vi "RFmx_Meas_Settings_SeqMode.vi"(7 "RFmx_Setting":T1={"Center Frequency (Hz)"=0.0, "Reference Level (dBm)"=0.0, "External Attenuation (dB)"=0.0, "ACP:Offset Frequency (Hz)"=[], "ACP:Integration Bandwidth (Hz)"=[], "CCDF:Threshold Level (dB or dBm)"=0.0, "CHP:Integration Bandwidth (Hz)"=0.0, "Fcnt:Threshold Level (dB or dBm)"=0.0, "OBW:Bandwidth Percentage (%)"=0.0, "Spectrum:Span (Hz)"=20000000.0, "TXP:Measurement Interval (s)"=0.0, "IQ:Bandwidth (Hz)"=1000000.0} {"IQ:Bandwidth (Hz)" format="%#_13p"; "TXP:Measurement Interval (s)" format="%#_6p"; "Spectrum:Span (Hz)" format="%#_13p"; "OBW:Bandwidth Percentage (%)" format="%#_6p"; "Fcnt:Threshold Level (dB or dBm)" format="%#_6p"; "CHP:Integration Bandwidth (Hz)" format="%#_6p"; "CCDF:Threshold Level (dB or dBm)" format="%#_6p"; "ACP:Integration Bandwidth (Hz)" format="%#_6p"; "ACP:Offset Frequency (Hz)" format="%#_6p"; "External Attenuation (dB)" format="%#_6p"; "Reference Level (dBm)" format="%#_6p"; "Center Frequency (Hz)" format="%#_6p"}, 8 "error in":errorcluster, 9 "Selector Strings":string[](array[string]), 10 "Measurements":T2(array[ring]), 11 "Instrument Handle in":refnum<k21>) -> (0 "error out":errorcluster, 3 "Instrument Handle out":refnum<k21>)   [LabVIEW 2014]
panel:
  # "클러스터 하나로 만들어야 함"
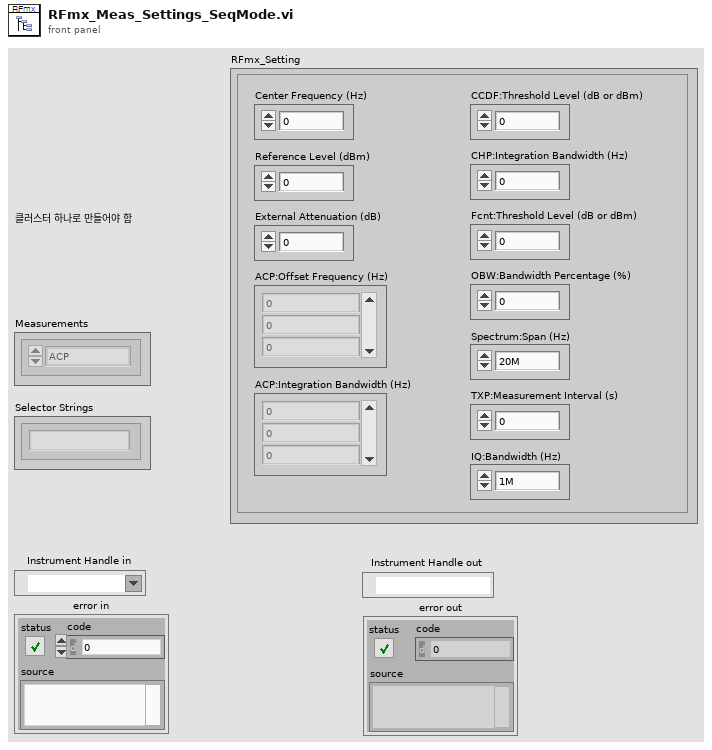
[diagram p1: front panel]
types:
  T1 = cluster{"Center Frequency (Hz)":dbl, "Reference Level (dBm)":dbl, "External Attenuation (dB)":dbl, "ACP:Offset Frequency (Hz)":dbl[], "ACP:Integration Bandwidth (Hz)":dbl[], "CCDF:Threshold Level (dB or dBm)":dbl, "CHP:Integration Bandwidth (Hz)":dbl, "Fcnt:Threshold Level (dB or dBm)":dbl, "OBW:Bandwidth Percentage (%)":dbl, "Spectrum:Span (Hz)":dbl, "TXP:Measurement Interval (s)":dbl, "IQ:Bandwidth (Hz)":dbl}
  T2 = enum16{"ACP", "CCDF", "CHP", "FCnt", "Harmonics", "OBW", "SEM", "Spectrum", "Spur", "TXP", "AMPM", "DPD", "IQ"}[]
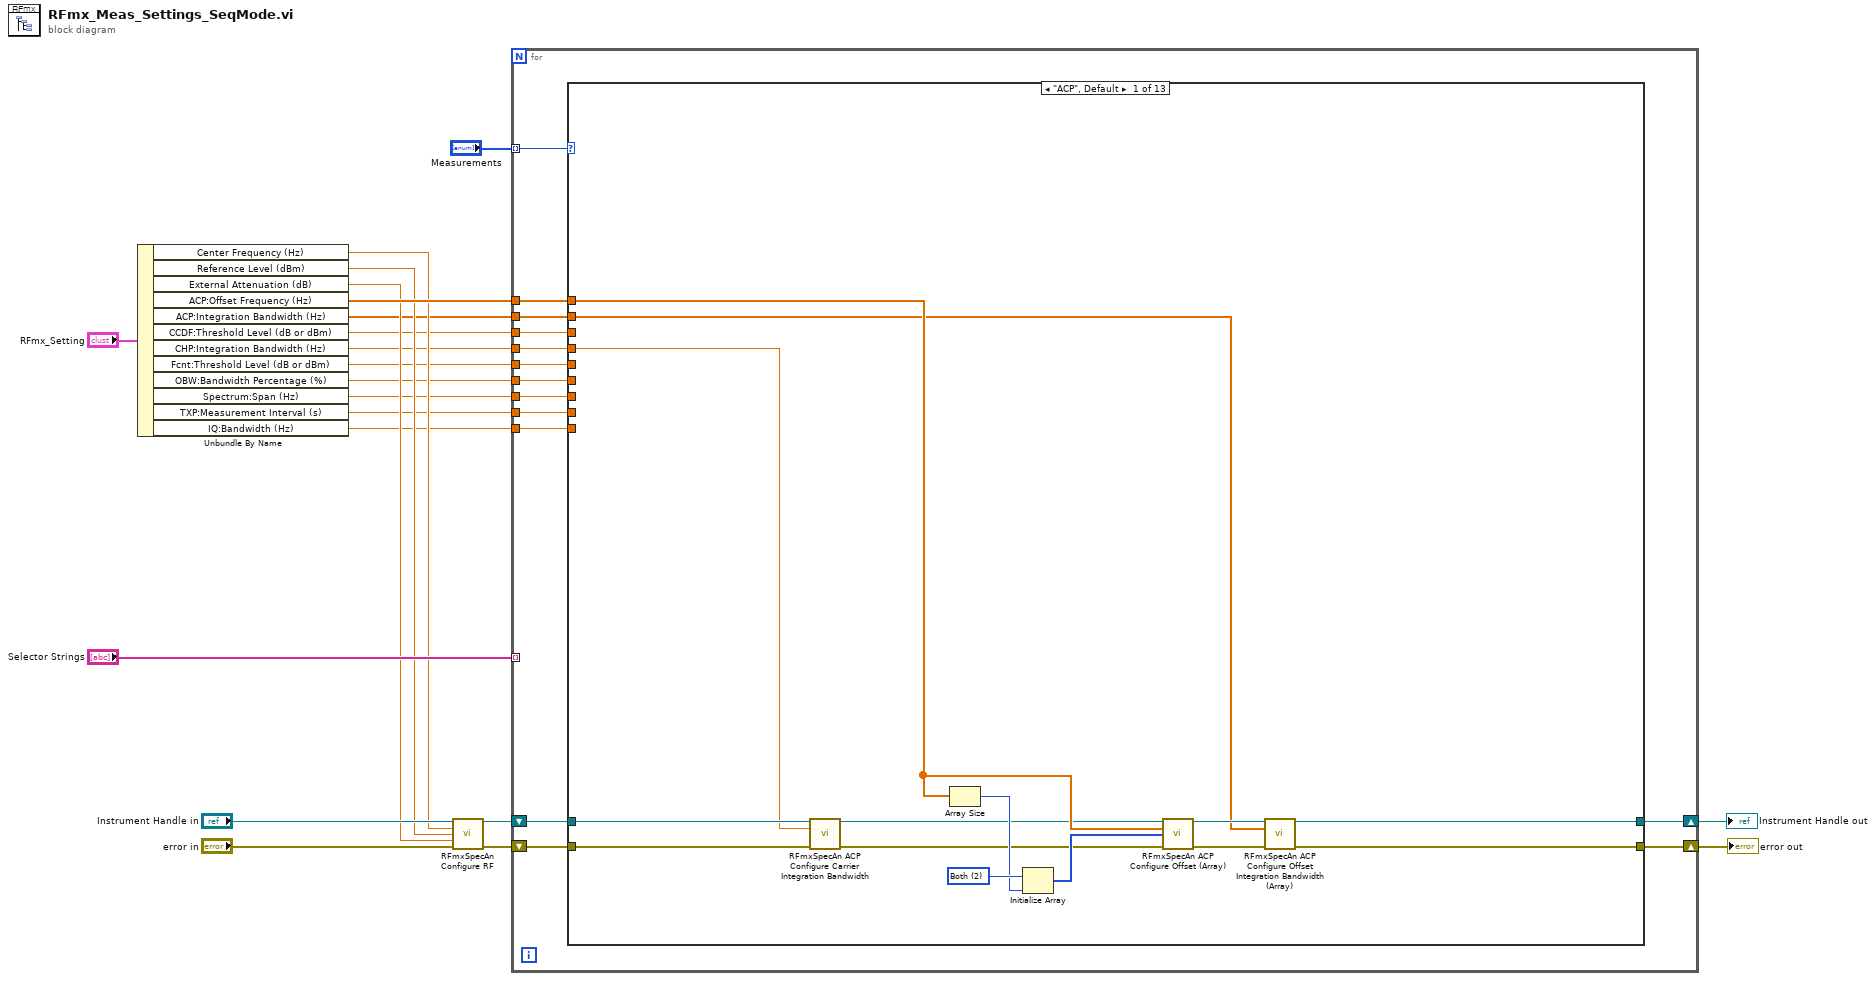
[diagram p0: block diagram]
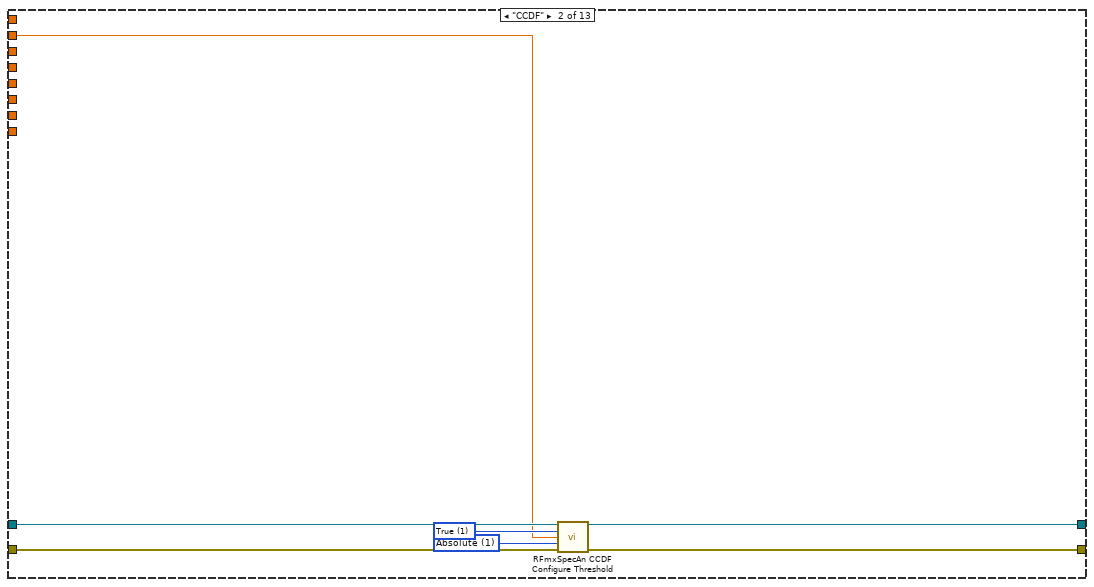
[diagram p2: hidden frame]
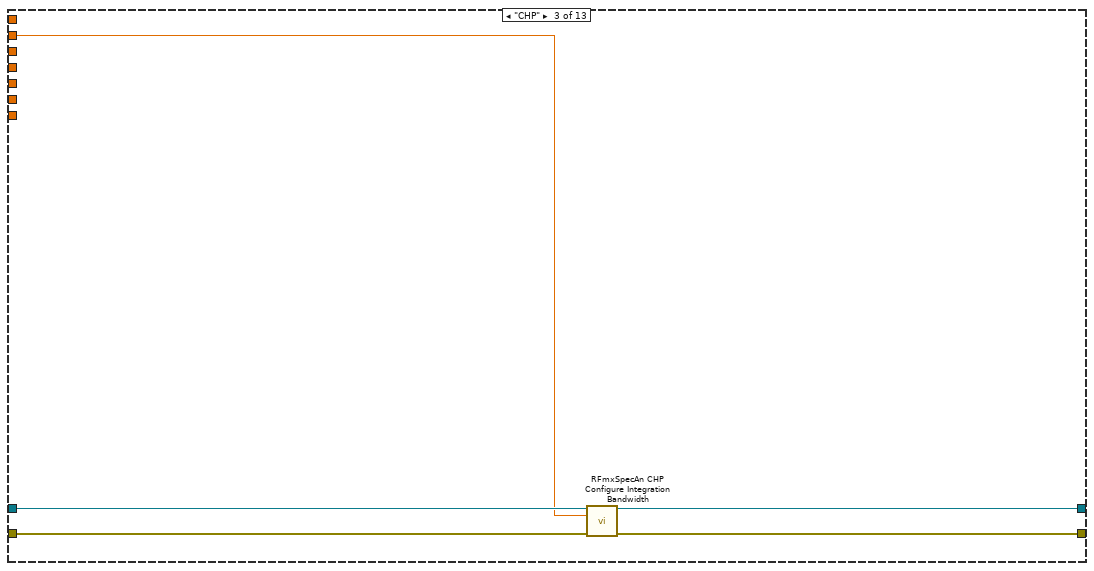
[diagram p3: hidden frame]
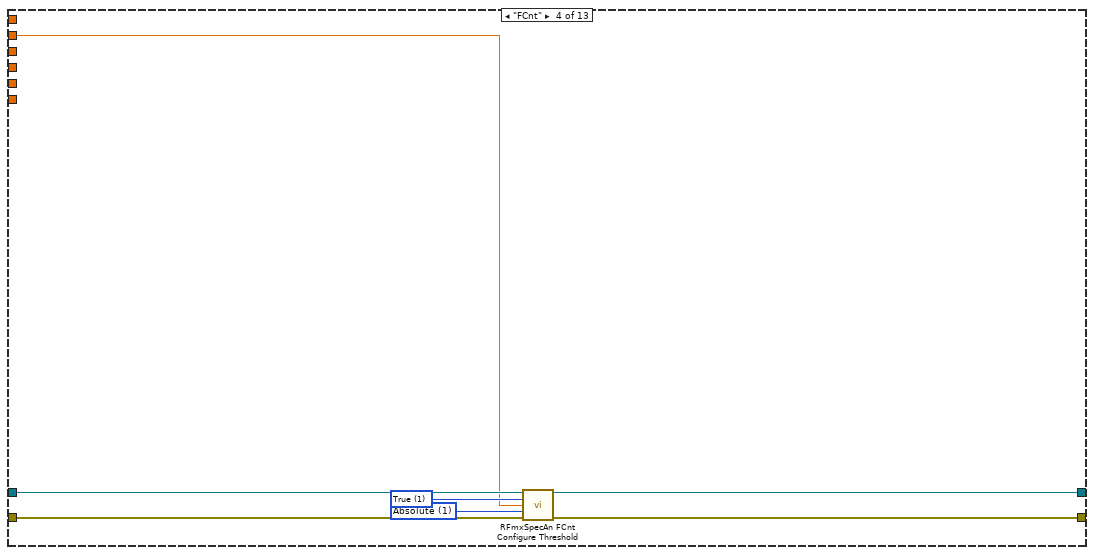
[diagram p4: hidden frame]
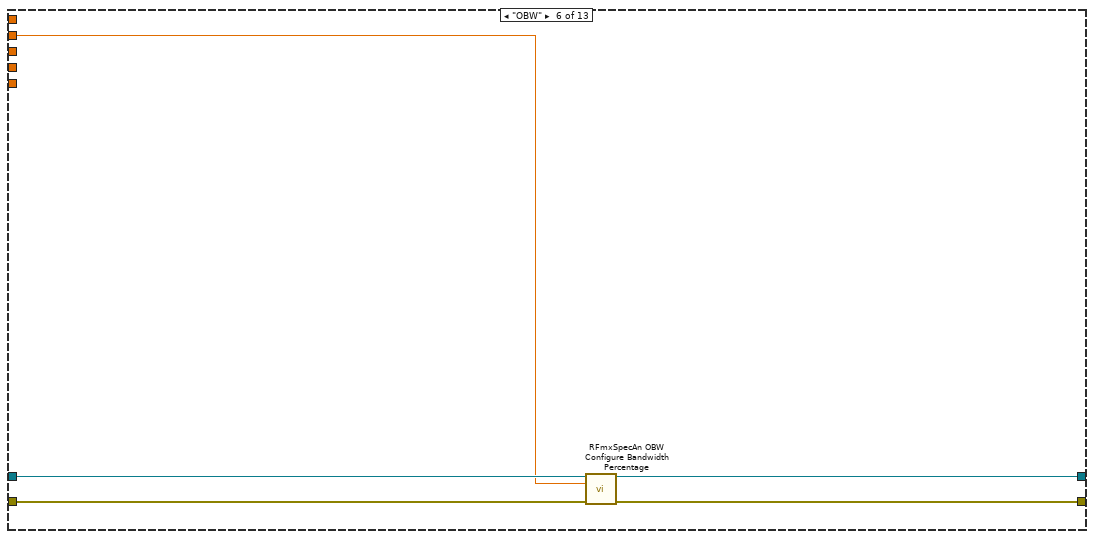
[diagram p6: hidden frame]
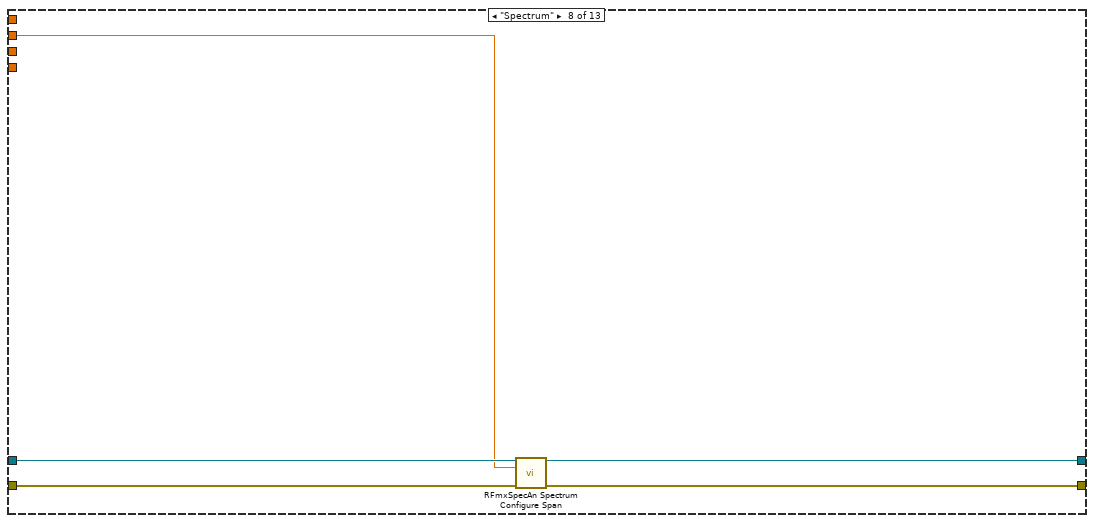
[diagram p8: hidden frame]
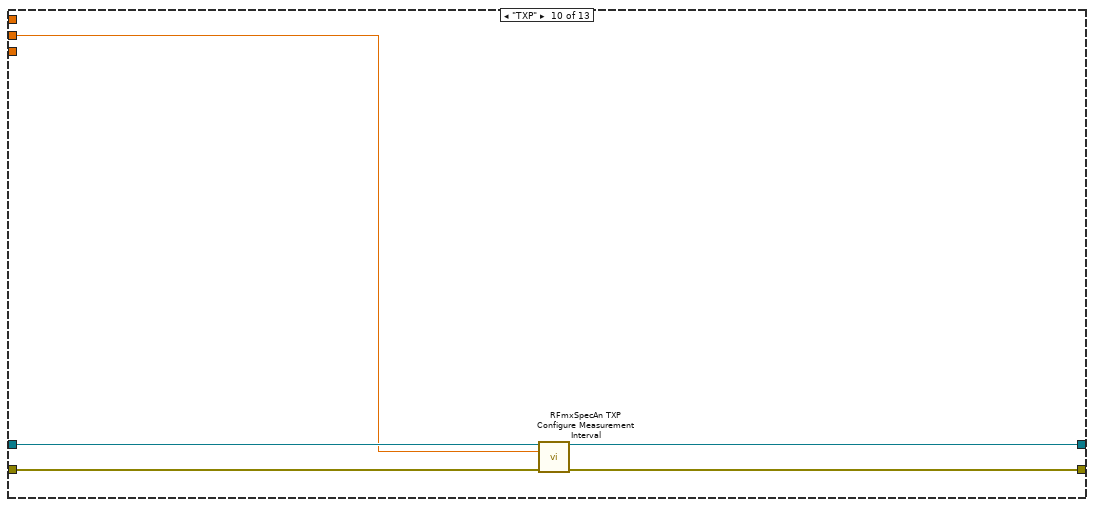
[diagram p10: hidden frame]
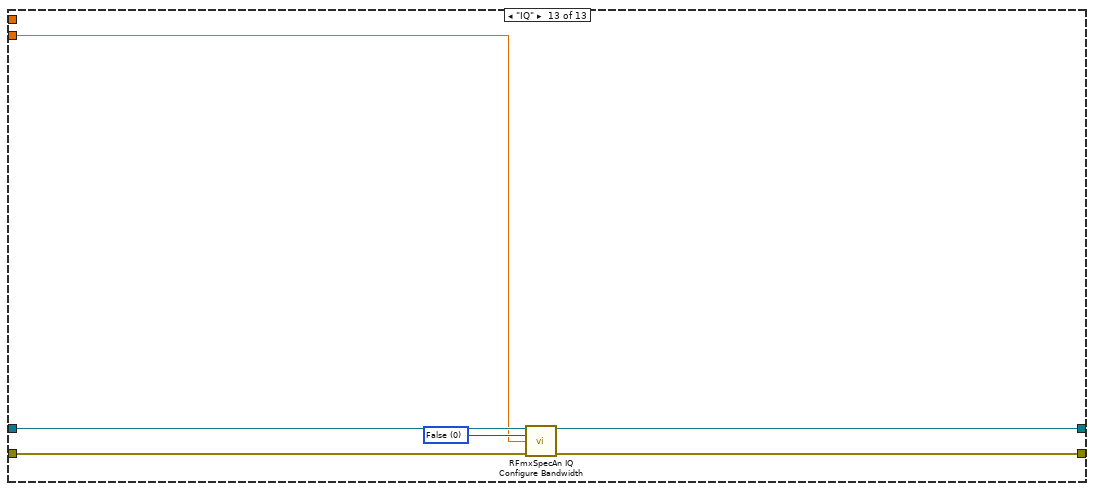
[diagram p13: hidden frame]
diagram:
  n1 = Unbundle By Name("RFmx_Setting") -> ("Center Frequency (Hz)"=w11:dbl, "Reference Level (dBm)"=w10:dbl, "External Attenuation (dB)"=w9:dbl, "ACP:Offset Frequency (Hz)"=w12:dbl[], "ACP:Integration Bandwidth (Hz)"=w8:dbl[], "CCDF:Threshold Level (dB or dBm)"=w7:dbl, "CHP:Integration Bandwidth (Hz)"=w6:dbl, "Fcnt:Threshold Level (dB or dBm)"=w5:dbl, "OBW:Bandwidth Percentage (%)"=w4:dbl, "Spectrum:Span (Hz)"=w3:dbl, "TXP:Measurement Interval (s)"=w2:dbl, "IQ:Bandwidth (Hz)"=w1:dbl)
  n2 = call <vilib>:"RFmxSpecAn Configure RF.vi"("Instrument Handle In"="Instrument Handle in", "Center Frequency (Hz)"=w11, "Reference Level (dBm)"=w10, "External Attenuation (dB)"=w9, "error in (no error)"="error in") -> ("Instrument Handle Out"=w15:refnum<k21>, "error out"=w14:errorcluster)  [unwired: 9 in]
  n3 = for {
    shift-right: [w35] -> w21
    shift-left: w15 -> [w33]
    shift-right: [w34] -> w20
    shift-left: w14 -> [w32]
    tunnel: "Measurements" -> [w31] mode=indexing
    tunnel: "Selector Strings" -> [_] mode=indexing
    tunnel: w12 -> [w30]
    tunnel: w8 -> [w29]
    tunnel: w7 -> [w28]
    tunnel: w6 -> [w27]
    tunnel: w5 -> [w26]
    tunnel: w4 -> [w25]
    tunnel: w3 -> [w24]
    tunnel: w2 -> [w23]
    tunnel: w1 -> [w22]
    n4 = case shown="\"ACP\", Default" w31 {
      tunnel: w33 -> [w40 w56 w61 w68 w69 w73 w77 w82 w84 w89 w91 w93 w96]
      tunnel: w32 -> [w39 w55 w60 w65 w70 w72 w76 w81 w83 w88 w90 w92 w95]
      tunnel: [w48 w53 w58 w67 w69 w75 w77 w80 w84 w86 w91 w93 w99] -> w35
      tunnel: [w47 w54 w59 w66 w70 w74 w76 w79 w83 w87 w90 w92 w98] -> w34
      tunnel: w30 -> [w42 _ _ _ _ _ _ _ _ _ _ _ _]
      tunnel: w29 -> [w41 _ _ _ _ _ _ _ _ _ _ _ _]
      tunnel: w28 -> [_ w50 _ _ _ _ _ _ _ _ _ _ _]
      tunnel: w27 -> [w36 _ w57 _ _ _ _ _ _ _ _ _ _]
      tunnel: w26 -> [_ _ _ w62 _ _ _ _ _ _ _ _ _]
      tunnel: w25 -> [_ _ _ _ _ w71 _ _ _ _ _ _ _]
      tunnel: w24 -> [_ _ _ _ _ _ _ w78 _ _ _ _ _]
      tunnel: w23 -> [_ _ _ _ _ _ _ _ _ w85 _ _ _]
      tunnel: w22 -> [_ _ _ _ _ _ _ _ _ _ _ _ w94]
      frame "ACP", Default {
        w45 = 2 items=["Neg", "Pos", "Both"] ("Offset Frequency Sideband")
        n5 = call <vilib>:"RFmxSpecAn ACP Configure Carrier Integration Bandwidth.vi"("Instrument Handle In"=w40, "Integration Bandwidth (Hz)"=w36, "error in (no error)"=w39) -> ("Instrument Handle Out"=w37:refnum<k21>, "error out"=w38:errorcluster)  [unwired: 11 in]
        n6 = Array Size(array=w42) -> (size(s)=w44:i32)
        n7 = Initialize Array(w45, w44) -> (w43:i32[])
        n8 = call <vilib>:"RFmxSpecAn ACP Configure Offset (Array).vi"("Instrument Handle In"=w37, "Offset Frequency (Hz)"=w42, "Offset Sideband"=w43, "error in (no error)"=w38) -> ("Instrument Handle Out"=w49:refnum<k21>, "error out"=w46:errorcluster)  [unwired: 10 in]
        n9 = call <vilib>:"RFmxSpecAn ACP Configure Offset Integration Bandwidth (Array).vi"("Instrument Handle In"=w49, "Integration Bandwidth (Hz)"=w41, "error in (no error)"=w46) -> ("Instrument Handle Out"=w48:refnum<k21>, "error out"=w47:errorcluster)  [unwired: 11 in]
      }
      frame "CCDF" {
        w51 = 1 items=["Relative", "Absolute"] ("Threshold Type")
        w52 = 1 items=["False", "True"] ("Threshold Enabled")
        n10 = call <vilib>:"RFmxSpecAn CCDF Configure Threshold.vi"("Instrument Handle In"=w56, "Threshold Enabled"=w52, "Threshold Level (dB or dBm)"=w50, "Threshold Type"=w51, "error in (no error)"=w55) -> ("Instrument Handle Out"=w53:refnum<k21>, "error out"=w54:errorcluster)  [unwired: 9 in]
      }
      frame "CHP" {
        n11 = call <vilib>:"RFmxSpecAn CHP Configure Integration Bandwidth.vi"("Instrument Handle In"=w61, "Integration Bandwidth (Hz)"=w57, "error in (no error)"=w60) -> ("Instrument Handle Out"=w58:refnum<k21>, "error out"=w59:errorcluster)  [unwired: 11 in]
      }
      frame "FCnt" {
        w63 = 1 items=["Relative", "Absolute"] ("Threshold Type")
        w64 = 1 items=["False", "True"] ("Threshold Enabled")
        n12 = call <vilib>:"RFmxSpecAn FCnt Configure Threshold.vi"("Instrument Handle In"=w68, "Threshold Enabled"=w64, "Threshold Level (dB or dBm)"=w62, "Threshold Type"=w63, "error in (no error)"=w65) -> ("Instrument Handle Out"=w67:refnum<k21>, "error out"=w66:errorcluster)  [unwired: 9 in]
      }
      frame "Harmonics" {
        # "Harmonics는 5665, 5668R에만 적용 가능함"
      }
      frame "OBW" {
        n13 = call <vilib>:"RFmxSpecAn OBW Configure Bandwidth Percentage.vi"("Instrument Handle In"=w73, "Bandwidth Percentage (%)"=w71, "error in (no error)"=w72) -> ("Instrument Handle Out"=w75:refnum<k21>, "error out"=w74:errorcluster)  [unwired: 11 in]
      }
      frame "SEM" {
        # "적용해야할 부분이 많으므로 다음에 추가할 예정"
      }
      frame "Spectrum" {
        n14 = call <vilib>:"RFmxSpecAn Spectrum Configure Span.vi"("Instrument Handle In"=w82, "Span (Hz)"=w78, "error in (no error)"=w81) -> ("Instrument Handle Out"=w80:refnum<k21>, "error out"=w79:errorcluster)  [unwired: 11 in]
      }
      frame "Spur" {
        # "Spur는 5665, 5668R에만 적용 가능함"
      }
      frame "TXP" {
        n15 = call <vilib>:"RFmxSpecAn TXP Configure Measurement Interval.vi"("Instrument Handle In"=w89, "Measurement Interval (s)"=w85, "error in (no error)"=w88) -> ("Instrument Handle Out"=w86:refnum<k21>, "error out"=w87:errorcluster)  [unwired: 11 in]
      }
      frame "AMPM" {
        # "적용해야할 부분이 많으므로 다음에 추가할 예정"
      }
      frame "DPD" {
        # "적용해야할 부분이 많으므로 다음에 추가할 예정"
      }
      frame "IQ" {
        w97 = 0 items=["False", "True"] ("Bandwidth Auto")
        n16 = call <vilib>:"RFmxSpecAn IQ Configure Bandwidth.vi"("Instrument Handle In"=w96, "Bandwidth Auto"=w97, "Bandwidth (Hz)"=w94, "error in (no error)"=w95) -> ("Instrument Handle Out"=w99:refnum<k21>, "error out"=w98:errorcluster)  [unwired: 10 in]
      }
    }
  }
  "Instrument Handle out" <- w21
  "error out" <- w20
